vi "Verify DAQ_RIO change.vi"(11 "RIO? in":bool) -> (3 "RIO? out":bool)   [LabVIEW 2013]
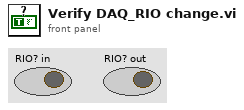
[diagram p1: front panel]
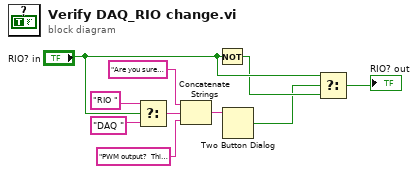
[diagram p0: block diagram]
diagram:
  n1 = Select(t="RIO ", s="RIO? in", f="DAQ ") -> (s? t:f=w7:string)
  n2 = Concatenate Strings("Are you sure you want to change this channel binding to " ("string"), w7, "PWM output?  This will change the required duty cycle format and remove any existing channel binding." ("string")) -> (w3:string)
  n3 = Not(x="RIO? in") -> (.not. x?=w8:bool)
  n4 = Two Button Dialog(message=w3) -> (T button?=w4:bool)  [unwired: 2 in]
  n5 = Select(t="RIO? in", s=w4, f=w8) -> (s? t:f=→"RIO? out":bool)
